vi "GetNodeMenuOptions.vi"(0 "reference in":refnum<class "InterfaceNode.lvclass">, 1 "MousePos":T1 {"y" format="%.2f"; "x" format="%.2f"}, 5 "error in (no error)":errorcluster) -> (14 "reference out":refnum<class "InterfaceNode.lvclass">, 15 "MenuOptions":string[](array[string]), 19 "error out":errorcluster)   [LabVIEW 2020, in "InterfaceNode.lvclass"]
uses:
  <resource>/Framework/Providers/Open_GDS/UML/InterfaceNode_class/InterfaceNode.lvclass
  <resource>/Framework/Providers/Open_GDS/UML/General/Point/Point Point2D.ctl
  <resource>/Framework/Providers/Open_GDS/UML/ClassNode_class/ClassNode.lvclass
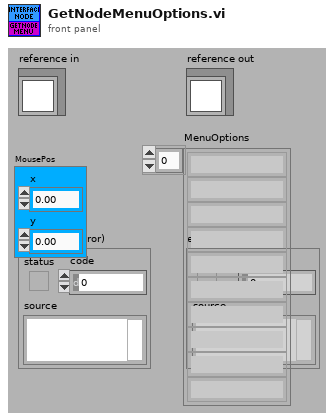
[diagram p1: front panel]
types:
  T1 = typedef "Point Point2D.ctl" = cluster{"x":dbl, "y":dbl}
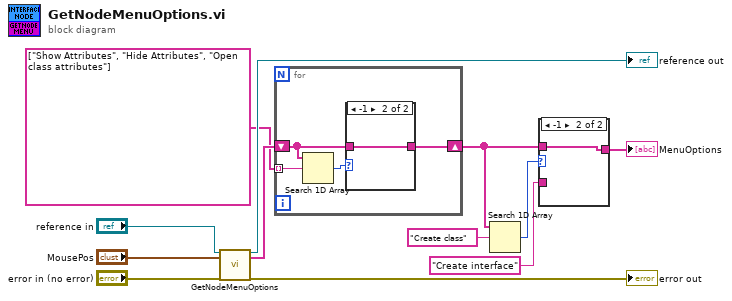
[diagram p0: block diagram]
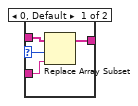
[diagram p2: hidden frame]
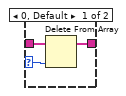
[diagram p3: hidden frame]
diagram:
  n1 = call-parent "GetNodeMenuOptions.vi"("reference"="reference in", "MousePos"="MousePos", "error in (no error)"="error in (no error)") -> ("reference out"=→"reference out":refnum<class "InterfaceNode.lvclass">, "MenuOptions"=w7:string[], "error out"=→"error out":errorcluster)  [unwired: 14 in]
  n2 = for {
    shift-right: [w13] -> w3
    shift-left: w7 -> [w14]
    tunnel: string[] ["Show Attributes", "Hide Attributes", "Open class attributes"] ("element") -> [w16] mode=indexing
    n3 = Search 1D Array(1D array=w14, element=w16) -> (index of element=w15:i32)  [unwired: 1 in]
    n4 = case shown="-1" w15 {
      selector: w15 -> [w18 _]
      tunnel: w14 -> [w19 w20]
      tunnel: [w17 w20] -> w13
      frame 0, Default {
        n5 = Delete From Array(array=w19, index=w18) -> (array with subset deleted=w17:string[])  [unwired: 1 in, 1 out]
      }
      frame -1 {
      }
    }
  }
  n6 = Search 1D Array(1D array=w3, element="Create class") -> (index of element=w4:i32)  [unwired: 1 in]
  n7 = case shown="-1" w4 {
    selector: w4 -> [w23 _]
    tunnel: w3 -> [w24 w25]
    tunnel: "Create interface" ("element") -> [w22 _]
    tunnel: [w21 w25] -> w1
    frame 0, Default {
      n8 = Replace Array Subset(array=w24, new element=w22, index=w23) -> (w21:string[])
    }
    frame -1 {
    }
  }
  "MenuOptions" <- w1
